vi "RGB Value Change.vi"(8 "error in (no error)":errorcluster, 11 "ColorSelector in":refnum<class "ColorSelector.lvclass">) -> (0 "error out":errorcluster, 3 "ColorSelector out":refnum<class "ColorSelector.lvclass">)   [LabVIEW 2015, in "ColorSelector.lvclass"]
doc: "This VI executes when the RGB values are changed. It does the math necessary to find and highlight the correct Grey and Color.\n<b> </b> <b> </b>\n©2017 Q Software Innovations, LLC (QSI)\nwritten by Quentin Alldredge\nproduced in LabVIEW 2015\n\nsupport@qsoftwareinnovations.com\nwww.qsoftwareinnovations.com\n\nAll rights reserved.\n\nRedistribution and use in source and binary forms, with or without modification, are permitted provided that the following conditions are met:\n\n * Redistributions of source code must retain the above copyright notice, this list of conditions and the following disclaimer.\n * Redistributions in binary form must reproduce the above copyright notice, this list of conditions and the following disclaimer in the documentation and/or other materials provided with the distribution.\n * Neither the name of Q Software Innovations, LLC. nor the names of its contributors may be used to endorse or promote products derived from this software without specific prior written permission.\n\nTHIS SOFTWARE IS PROVIDED BY THE COPYRIGHT HOLDERS AND CONTRIBUTORS \"AS IS\" AND ANY EXPRESS OR IMPLIED WARRANTIES, INCLUDING, BUT NOT LIMITED TO, THE IMPLIED WARRANTIES OF MERCHANTABILITY AND FITNESS FOR A PARTICULAR PURPOSE ARE DISCLAIMED. IN NO EVENT SHALL THE COPYRIGHT OWNER OR CONTRIBUTORS BE LIABLE FOR ANY DIRECT, INDIRECT, INCIDENTAL, SPECIAL, EXEMPLARY, OR CONSEQUENTIAL DAMAGES (INCLUDING, BUT NOT LIMITED TO, PROCUREMENT OF SUBSTITUTE GOODS OR SERVICES; LOSS OF USE, DATA, OR PROFITS; OR BUSINESS INTERRUPTION) HOWEVER CAUSED AND ON ANY THEORY OF LIABILITY, WHETHER IN CONTRACT, STRICT LIABILITY, OR TORT (INCLUDING NEGLIGENCE OR OTHERWISE) ARISING IN ANY WAY OUT OF THE USE OF THIS SOFTWARE, EVEN IF ADVISED OF THE POSSIBILITY OF SUCH DAMAGE."
uses:
  ColorSelector.lvclass
  ColorSelector.lvclass/ColorSelector.ctl
  <vilib>/Analysis/NI_AALPro.lvlib
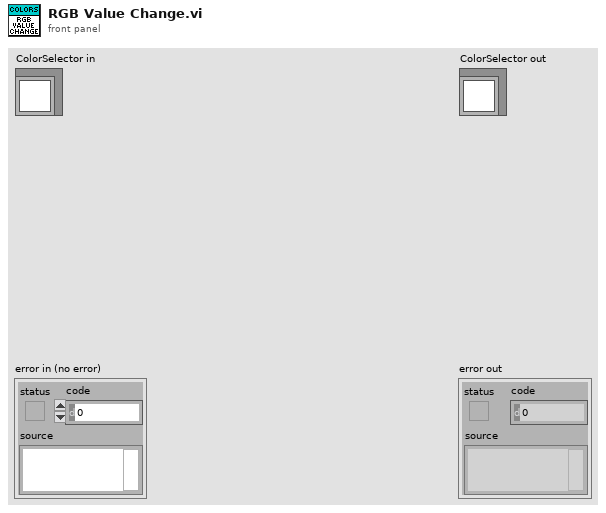
[diagram p1: front panel]
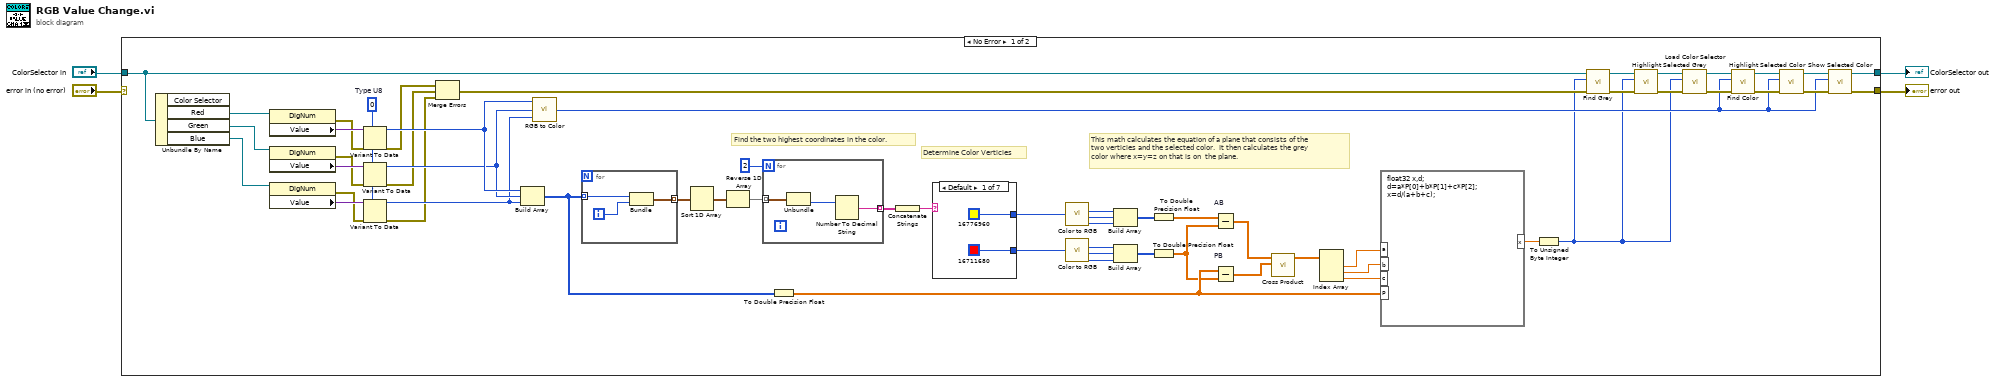
[diagram p0: block diagram]
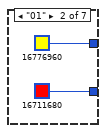
[diagram p2: hidden frame]
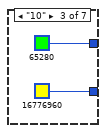
[diagram p3: hidden frame]
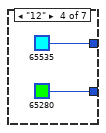
[diagram p4: hidden frame]
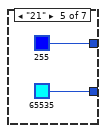
[diagram p5: hidden frame]
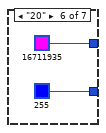
[diagram p6: hidden frame]
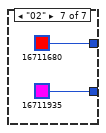
[diagram p7: hidden frame]
diagram:
  n1 = case shown="No Error" "error in (no error)" {
    selector: "error in (no error)" -> [_ w85]
    tunnel: [w11 w85] -> w3
    tunnel: [w34 w84] -> w1
    tunnel: "ColorSelector in" -> [w10 w84]
    frame No Error {
      w18 = u8 0  # Type U8
      # "Determine Color Verticies"
      # "This math calculates the equation of a plane that consists of the \ntwo verticies and the selected color.  It then calculates the grey \ncolor where x=y=z on that is on  the plane."
      # "Find the two highest coordinates in the color."
      n2 = Unbundle By Name(w10) -> ("Red"=w24:refnum<vi>, "Green"=w22:refnum<vi>, "Blue"=w21:refnum<vi>)  [unwired: 1 out]
      n3 = property class="DigNum"(reference=w24) -> (error out=w17:errorcluster, "Value"=w23:variant)  [unwired: 1 in, 1 out]
      n4 = property class="DigNum"(reference=w22) -> (error out=w16:errorcluster, "Value"=w20:variant)  [unwired: 1 in, 1 out]
      n5 = property class="DigNum"(reference=w21) -> (error out=w15:errorcluster, "Value"=w19:variant)  [unwired: 1 in, 1 out]
      n6 = Variant To Data(error in=w17, type=w18, Variant=w23) -> (data=w27:u8, error out=w14:errorcluster)
      n7 = Variant To Data(error in=w16, type=w18, Variant=w20) -> (data=w26:u8, error out=w13:errorcluster)
      n8 = Variant To Data(error in=w15, type=w18, Variant=w19) -> (data=w25:u8, error out=w12:errorcluster)
      n9 = Merge Errors(w14, w13, w12) -> (w8:errorcluster)
      n10 = Build Array(w27, w26, w25) -> (w62:u8[])
      n11 = call <vilib>:"RGB to Color.vi"("B"=w25, "G"=w26, "R"=w27) -> ("Color"=w6:u32)
      n12 = for {
        tunnel: w62 -> [w80] mode=indexing
        tunnel: [w78] -> w61 mode=indexing
        i -> [w79]
        n13 = Bundle("Type U8"=w80, w79) -> (w78:cluster{"Type U8":u8, i32})  [unwired: 1 in]
      }
      n14 = Sort 1D Array(array=w61) -> (sorted array=w59:cluster{"Type U8":u8, i32}[])
      n15 = Reverse 1D Array(array=w59) -> (reversed array=w58:cluster{"Type U8":u8, i32}[])
      n16 = for {
        N: 2 -> [_]
        tunnel: w58 -> [w83] mode=indexing
        tunnel: [w81] -> w57 mode=indexing
        n17 = Unbundle(w83) -> (w82:i32)  [unwired: 1 out]
        n18 = Number To Decimal String(number=w82) -> (decimal integer string=w81:string)  [unwired: 1 in]
      }
      n19 = To Double Precision Float(number=w62) -> (double precision float=w63:dbl[])
      n20 = Concatenate Strings(w57) -> (w56:string)
      n21 = case shown="Default" w56 {
        tunnel: [u32 16711680 u32 16711680 u32 16776960 u32 65280 u32 65535 u32 255 u32 16711935] -> w55
        tunnel: [u32 16776960 u32 16776960 u32 65280 u32 65535 u32 255 u32 16711935 u32 16711680] -> w54
        frame Default {
        }
        frame "01" {
        }
        frame "10" {
        }
        frame "12" {
        }
        frame "21" {
        }
        frame "20" {
        }
        frame "02" {
        }
      }
      n22 = call <vilib>:"Color to RGB.vi"("Color"=w54) -> ("R"=w45:u8, "G"=w51:u8, "B"=w50:u8)  [unwired: 1 out]
      n23 = call <vilib>:"Color to RGB.vi"("Color"=w55) -> ("R"=w46:u8, "G"=w53:u8, "B"=w52:u8)  [unwired: 1 out]
      n24 = Build Array(w45, w51, w50) -> (w44:u8[])
      n25 = Build Array(w46, w53, w52) -> (w43:u8[])
      n26 = To Double Precision Float(number=w44) -> (double precision float=w38:dbl[])
      n27 = To Double Precision Float(number=w43) -> (double precision float=w39:dbl[])
      n28 = Subtract "AB"(x=w38, y=w39) -> (x-y=w40:dbl[])
      n29 = Subtract "PB"(x=w63, y=w39) -> (x-y=w42:dbl[])
      n30 = call <vilib>:"Cross Product.vi"("B Vector"=w42, "A Vector"=w40) -> ("Cross Product"=w41:dbl[])  [unwired: 8 in, 1 out]
      n31 = Index Array(array=w41) -> (element #1=w49:dbl, element #2=w48:dbl, element #3=w47:dbl)  [unwired: 3 in]
      n32 = formula code="float32 x,d;\nd=a*P[0]+b*P[1]+c*P[2];\nx=d/(a+b+c);"("a"=w49, "b"=w48, "c"=w47, "P"=w63) -> ("x"=w37:sgl)
      n33 = To Unsigned Byte Integer(number=w37) -> (unsigned 8bit integer=w5:u8)
      n34 = call "Find Grey.vi"("error in (no error)"=w8, "Grey Index (0-255)"=w5, "ColorSelector in"=w10) -> ("error out"=w7:errorcluster, "ColorSelector out"=w9:refnum<class "ColorSelector.lvclass">)  [unwired: 7 in]
      n35 = call "Highlight Selected Grey.vi"("error in (no error)"=w7, "Grayscale Index (0-255)"=w5, "ColorSelector in"=w9) -> ("error out"=w33:errorcluster, "ColorSelector (dup)"=w36:refnum<class "ColorSelector.lvclass">)  [unwired: 7 in]
      n36 = call "Load Color Selector.vi"("error in (no error)"=w33, "Grayscale Index (0-255)"=w5, "ColorSelector in"=w36) -> ("error out"=w29:errorcluster, "ColorSelector out"=w31:refnum<class "ColorSelector.lvclass">)  [unwired: 7 in]
      n37 = call "Find Color.vi"("error in (no error)"=w29, "Color Selected"=w6, "ColorSelector in"=w31) -> ("error out"=w28:errorcluster, "ColorSelector out"=w30:refnum<class "ColorSelector.lvclass">)  [unwired: 7 in]
      n38 = call "Highlight Selected Color.vi"("error in (no error)"=w28, "Selected Color"=w6, "ColorSelector in"=w30) -> ("error out"=w32:errorcluster, "ColorSelector (dup)"=w35:refnum<class "ColorSelector.lvclass">)  [unwired: 7 in]
      n39 = call "Show Selected Color.vi"("error in (no error)"=w32, "Selected Color"=w6, "ColorSelector in"=w35) -> ("error out"=w11:errorcluster, "ColorSelector (dup)"=w34:refnum<class "ColorSelector.lvclass">)  [unwired: 7 in]
    }
    frame Error {
    }
  }
  "error out" <- w3
  "ColorSelector out" <- w1
